vi "Create Chunk (subVI).vi"(8 "error in (no error)":errorcluster, 10 "Byte Array":u8[](array[numeric])) -> (0 "error out":errorcluster, 1 "size string":string, 2 "Chunk String":string)   [LabVIEW 2015]
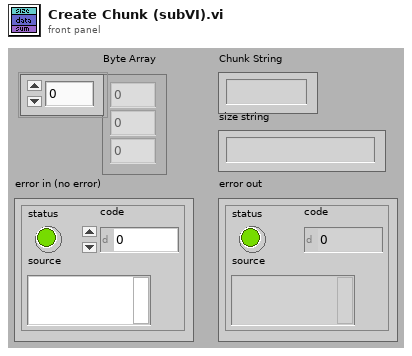
[diagram p1: front panel]
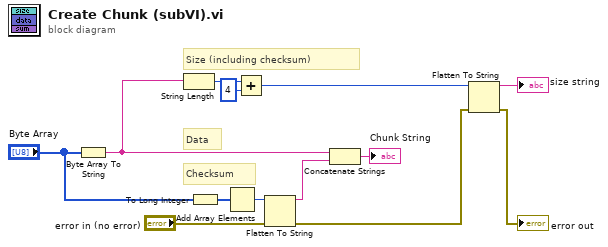
[diagram p0: block diagram]
diagram:
  # "Checksum"
  # "Data"
  # "Size (including checksum)"
  n1 = Byte Array To String(unsigned byte array="Byte Array") -> (string=w6:string)
  n2 = String Length(string=w6) -> (length=w9:i32)
  n3 = To Long Integer(number="Byte Array") -> (32bit integer=w13:i32[])
  n4 = Add Array Elements(numeric array=w13) -> (sum=w12:i32)
  n5 = Add(x=w9, y=4) -> (x+y=w8:i32)
  n6 = Flatten To String(anything=w12, error in (no error)="error in (no error)") -> (data string=w11:string, error out=w2:errorcluster)  [unwired: 3 out]
  n7 = Concatenate Strings(w6, w11) -> (→"Chunk String":string)
  n8 = Flatten To String(anything=w8, error in (no error)=w2) -> (data string=→"size string":string, error out=→"error out":errorcluster)  [unwired: 3 out]
